vi "Agilent SNA Set Channel.vi"(7 "Agilent SNA & SWP":T2, 8 "error in (no error)":errorcluster, 10 "Channel":i8=1 min=1 max=99 step=1, 11 "VISA Resource Names":T1) -> (0 "error out":errorcluster, 3 "dup VISA Resource Names":T1)   [LabVIEW 2011]
uses:
  TypeDefs/Agilent SNA Instrument Info.ctl
  TypeDefs/Agilent SNA VISA.ctl
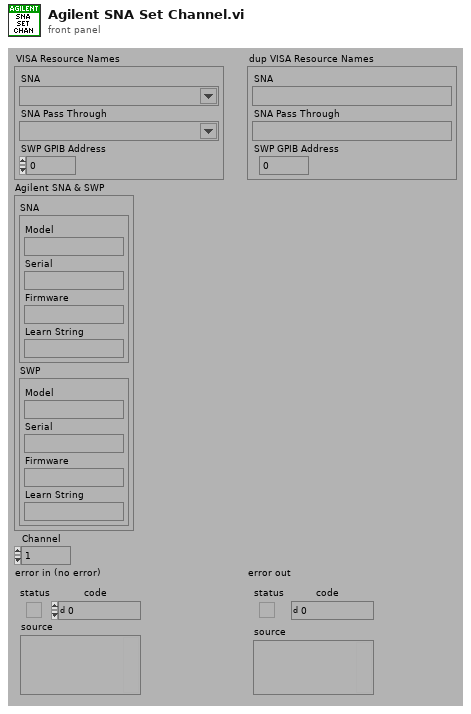
[diagram p1: front panel]
types:
  T1 = typedef "Agilent SNA VISA.ctl" = cluster{"SNA":refnum<visa-resource-name>, "SNA Pass Through":refnum<visa-resource-name>, "SWP GPIB Address":i32}
  T2 = typedef "Agilent SNA Instrument Info.ctl" = cluster{"SNA":cluster{"Model":string, "Serial":string, "Firmware":string, "Learn String":string}, "SWP":cluster{"Model":string, "Serial":string, "Firmware":string, "Learn String":string}}
  T3 = typedef "Agilent SNA Model.ctl" = enum16{"Not Supported", "8757X"}
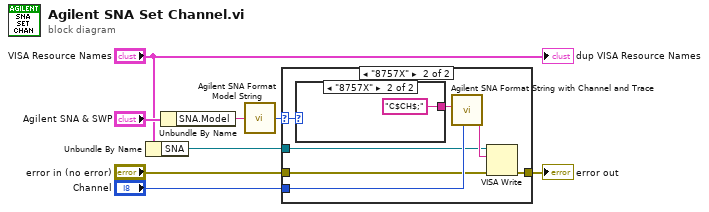
[diagram p0: block diagram]
diagram:
  n1 = Unbundle By Name("VISA Resource Names") -> ("SNA"=w1:refnum<visa-resource-name>)
  n2 = Unbundle By Name("Agilent SNA & SWP") -> ("SNA.Model"=w4:string)
  n3 = call "Agilent SNA Format Model String.vi"("Model String"=w4) -> ("Model"=w5:T3)
  n4 = case shown="\"8757X\"" w5 {
    selector: w5 -> [_ w12]
    tunnel: [w9 w16] -> w8
    tunnel: w1 -> [_ w11]
    tunnel: "error in (no error)" -> [w9 w10]
    tunnel: "Channel" -> [_ w13]
    frame "Not Supported" {
    }
    frame "8757X" {
      n5 = case shown="\"8757X\"" w12 {
        tunnel: [_ "C$CH$;"] -> w14
        frame "Not Supported" {
        }
        frame "8757X" {
        }
      }
      n6 = call "Agilent SNA Format String with Channel and Trace.vi"("Channel"=w13, "String"=w14) -> ("String Out"=w15:string)  [unwired: 1 in, 6 out]
      n7 = VISA Write(VISA resource name=w11, write buffer=w15, error in (no error)=w10) -> (error out=w16:errorcluster)  [unwired: 2 out]
    }
  }
  "error out" <- w8
  "dup VISA Resource Names" <- "VISA Resource Names"
